vi "Reload.vi"(8 "Error In":errorcluster, 11 "object in":refnum<class "WebView.lvclass">) -> (0 "Error Out":errorcluster, 3 "object out":refnum<class "WebView.lvclass">)   [LabVIEW 2024, in "WebView.lvclass"]
uses:
  WebView.lvclass
  WebView.lvclass/WebView.ctl
  <vilib>/sklein/WebView2/Libs/Microsoft.Web.WebView2.Core.dll
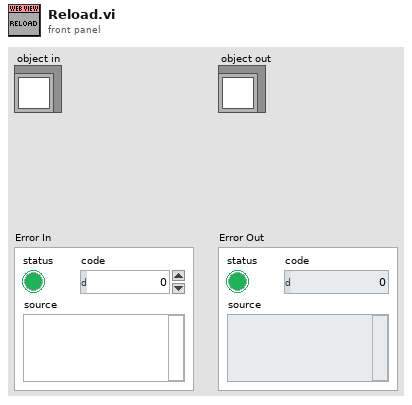
[diagram p1: front panel]
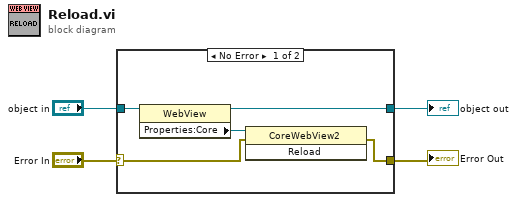
[diagram p0: block diagram]
diagram:
  n1 = case shown="No Error" "Error In" {
    selector: "Error In" -> [w6 w11]
    tunnel: [w5 w11] -> w3
    tunnel: [w8 w10] -> w1
    tunnel: "object in" -> [w9 w10]
    frame No Error {
      n2 = property class="WebView"(reference=w9) -> (reference out=w8:refnum<class "WebView.lvclass">, "Properties:Core"=w7:refnum<k24>)  [unwired: 1 in, 1 out]
      n3 = invoke class="CoreWebView2" method="Reload"(reference=w7, error in=w6) -> (error out=w5:errorcluster)  [unwired: 1 in, 2 out]
    }
    frame Error {
    }
  }
  "Error Out" <- w3
  "object out" <- w1
